vi "Get Cargo Capacity.vi"(8 "error in":errorcluster, 11 "truck":refnum<class "Truck.lvclass">) -> (0 "error out":errorcluster, 2 "cargo capacity":dbl)   [LabVIEW 2020, in "Truck.lvclass"]
doc: "This VI is an example of an override member VI. It returns the cargo capacity for the truck."
uses:
  Truck.lvclass
  Truck.lvclass/Truck.ctl
  Vehicle/Vehicle.lvclass
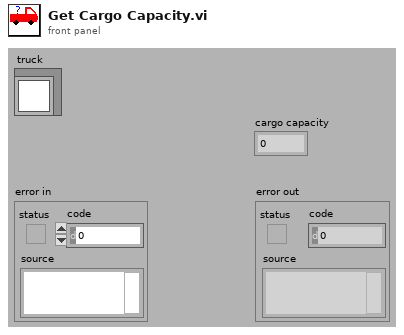
[diagram p1: front panel]
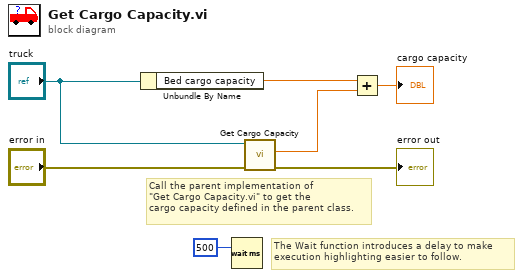
[diagram p0: block diagram]
diagram:
  # "Call the parent implementation of\n\"Get Cargo Capacity.vi\" to get the\ncargo capacity defined in the parent class."
  # "The Wait function introduces a delay to make\nexecution highlighting easier to follow."
  n1 = Unbundle By Name("truck") -> ("Bed cargo capacity"=w3:dbl)
  n2 = Wait (ms)(milliseconds to wait=u32 500) -> ()  [unwired: 1 out]
  n3 = call-parent "Get Cargo Capacity.vi"("error in"="error in", "vehicle"="truck") -> ("error out"=→"error out":errorcluster, "cargo capacity"=w2:dbl)  [unwired: 8 in]
  n4 = Add(x=w3, y=w2) -> (x+y=→"cargo capacity":dbl)
